vi "match serial.vi"() -> (2 "match?":bool, 3 "配置串口":string)   [LabVIEW 2016, in "DGUS.lvlib" / "DGUS.lvclass"]
uses:
  DGUS.lvclass
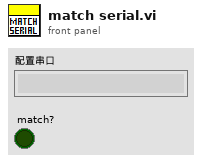
[diagram p1: front panel]
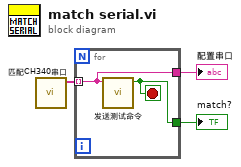
[diagram p0: block diagram]
diagram:
  n1 = call "匹配CH340串口.vi"() -> ("find list"=w1:string[])  [unwired: 11 in]
  n2 = for {
    tunnel: w1 -> [w5] mode=indexing
    tunnel: [w5] -> w3
    tunnel: [w4] -> w2
    stop <- w4 stop-if-true
    n3 = call "发送测试命令.vi"("VISA资源名称"=w5) -> ("match?"=w4:bool)  [unwired: 10 in]
  }
  "配置串口" <- w3
  "match?" <- w2
